vi "Build SPA command substring.vi"(0 "System no.":i32=1 min=1 max=4 step=1, 2 "Axes to set":string[](array[string]), 3 "Parameter values":dbl[](array[numeric]) format="%.6f", 4 "No. of digits":i16=4, 6 "Parameter number":i32[](array[numeric]), 7 "Parameter no. format \n(Decimal: FALSE)":bool, 8 "Parameter number (hex)":u32[](array[numeric]) format="%.0x", 9 "Parameter format \n(Num.: FALSE)":bool, 10 "Parameter strings":string[](array[string]), 11 "With space?":bool) -> (14 "SPA command substring":string)   [LabVIEW 2026]
doc: "This VI builds a command substring for the SPA command. No. of digits is the number of digits after the decimal point in the parameter value(s) that will be sent. Sub-VI for SPA.vi, CTO.vi, WTR.vi."
panel:
  # "This vi builds a command substring for the SPA command."
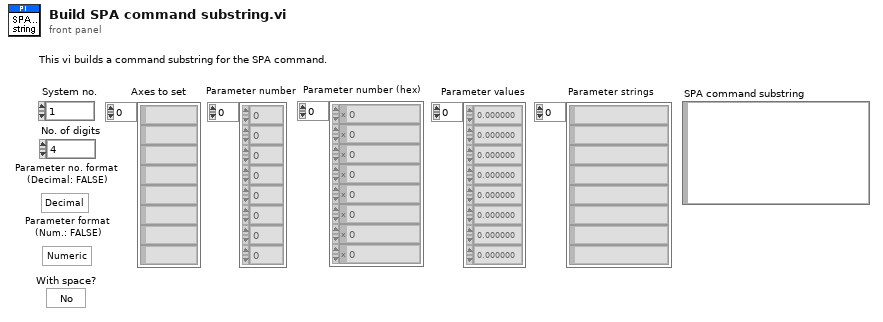
[diagram p1: front panel]
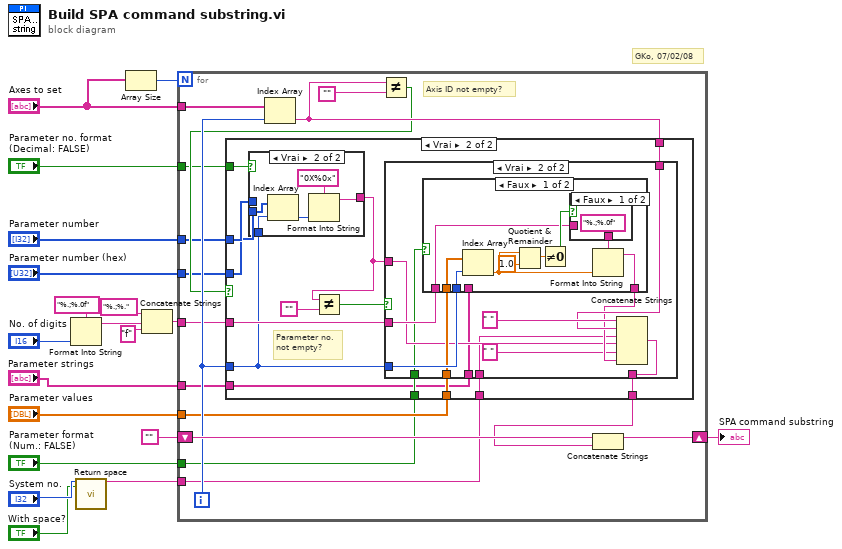
[diagram p0: block diagram]
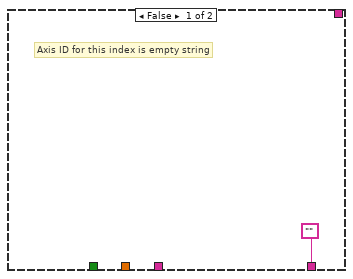
[diagram p2: hidden frame]
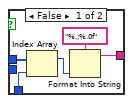
[diagram p3: hidden frame]
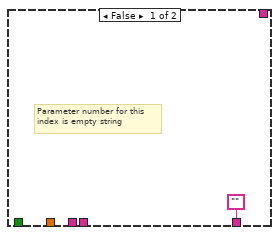
[diagram p4: hidden frame]
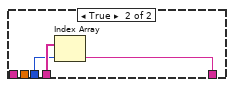
[diagram p6: hidden frame]
diagram:
  # "GKo, 07/02/08"
  n1 = Format Into String(format string="%.;%.0f" ("Format String"), "No. of digits") -> (resulting string=w4:string)  [unwired: 2 in, 1 out]
  n2 = call "Return space.vi"("System no."="System no.", "With space?"="With space?") -> ("String out"=w8:string)  [unwired: 17 out]
  n3 = Array Size(array="Axes to set") -> (size(s)=w16:i32)
  n4 = Concatenate Strings("%.;%." ("Format String"), w4, "f" ("Format String")) -> (w3:string)
  n5 = for {
    N: w16 -> [_]
    shift-right: [w34] -> w18
    shift-left: "" -> [w35]
    tunnel: "Parameter values" -> [w31]
    tunnel: w3 -> [w30]
    tunnel: "Axes to set" -> [w29]
    tunnel: "Parameter number" -> [w25]
    tunnel: "Parameter no. format \n(Decimal: FALSE)" -> [w24]
    tunnel: "Parameter number (hex)" -> [w23]
    tunnel: "Parameter format \n(Num.: FALSE)" -> [w22]
    tunnel: "Parameter strings" -> [w21]
    tunnel: w8 -> [w20]
    i -> [w32]
    # "Axis ID not empty?"
    n6 = Index Array(array=w29, index=w32) -> (element=w28:string)
    n7 = Not Equal?(x=w28, y="") -> (x != y?=w26:bool)
    n8 = case shown="Vrai" w26 {
      tunnel: ["" w50] -> w33
      tunnel: w32 -> [_ w45]
      tunnel: w31 -> [_ w49]
      tunnel: w30 -> [_ w48]
      tunnel: w28 -> [_ w47]
      tunnel: w25 -> [_ w46]
      tunnel: w24 -> [_ w41]
      tunnel: w23 -> [_ w40]
      tunnel: w22 -> [_ w39]
      tunnel: w21 -> [_ w38]
      tunnel: w20 -> [_ w37]
      frame False {
        # "Axis ID for this index is empty string"
      }
      frame True {
        # "Parameter no.\nnot empty?"
        n9 = case shown="Vrai" w41 {
          tunnel: w46 -> [w55 _]
          tunnel: w45 -> [w54 w56]
          tunnel: [w51 w58] -> w42
          tunnel: w40 -> [_ w57]
          frame False {
            n10 = Index Array(array=w55, index=w54) -> (element=w53:i32)
            n11 = Format Into String(format string="%.;%.0f" ("Format String"), w53) -> (resulting string=w51:string)  [unwired: 2 in, 1 out]
          }
          frame True {
            n12 = Index Array(array=w57, index=w56) -> (element=w60:u32)
            n13 = Format Into String(format string="0X%0x" ("Format String"), w60) -> (resulting string=w58:string)  [unwired: 2 in, 1 out]
          }
        }
        n14 = Not Equal?(x=w42, y="") -> (x != y?=w43:bool)
        n15 = case shown="Vrai" w43 {
          tunnel: ["" w73] -> w50
          tunnel: w45 -> [_ w72]
          tunnel: w49 -> [_ w71]
          tunnel: w48 -> [_ w70]
          tunnel: w47 -> [_ w68]
          tunnel: w42 -> [_ w65]
          tunnel: w39 -> [_ w64]
          tunnel: w38 -> [_ w63]
          tunnel: w37 -> [_ w62]
          frame False {
            # "Parameter number for this\nindex is empty string"
          }
          frame True {
            n16 = case shown="Faux" w64 {
              tunnel: w72 -> [w82 w86]
              tunnel: w71 -> [w81 _]
              tunnel: w70 -> [w75 _]
              tunnel: [w80 w85] -> w67
              tunnel: w63 -> [_ w87]
              frame False {
                n17 = Index Array(array=w81, index=w82) -> (element=w79:dbl)
                n18 = Quotient & Remainder(x=w79, y=1.0) -> (x-y*floor(x/y)=w77:dbl)  [unwired: 1 out]
                n19 = Not Equal To 0?(x=w77) -> (x != 0?=w76:bool)
                n20 = case shown="Faux" w76 {
                  tunnel: w75 -> [_ w84]
                  tunnel: ["%.;%.0f" ("Format String") w84] -> w74
                  frame False {
                  }
                  frame True {
                  }
                }
                n21 = Format Into String(format string=w74, w79) -> (resulting string=w80:string)  [unwired: 2 in, 1 out]
              }
              frame True {
                n22 = Index Array(array=w87, index=w86) -> (element=w85:string)
              }
            }
            n23 = Concatenate Strings(" " ("Substring"), w68, w62, w65, " " ("Substring"), w67) -> (w73:string)
          }
        }
      }
    }
    n24 = Concatenate Strings(w35, w33) -> (w34:string)
  }
  "SPA command substring" <- w18
